vi "Operate.vi"(0 "Add in":refnum<class "Add.lvclass">, 11 "error in (no error)":errorcluster) -> (4 "Add out":refnum<class "Add.lvclass">, 15 "error out":errorcluster)   [LabVIEW 2020, in "Add.lvclass"]
uses:
  Add.lvclass
  C:/Users/khishore.kumar/Khishore/labview_tips_2024/src/Assignment 25/Arithmetic Operations/Arithmetic Operations.lvclass
  Arithmetic Operations.lvclass/Arithmetic Operations.ctl
  Accessors/Read/Read A.vi
  Accessors/Read/Read B.vi
  Accessors/Write/Write C.vi
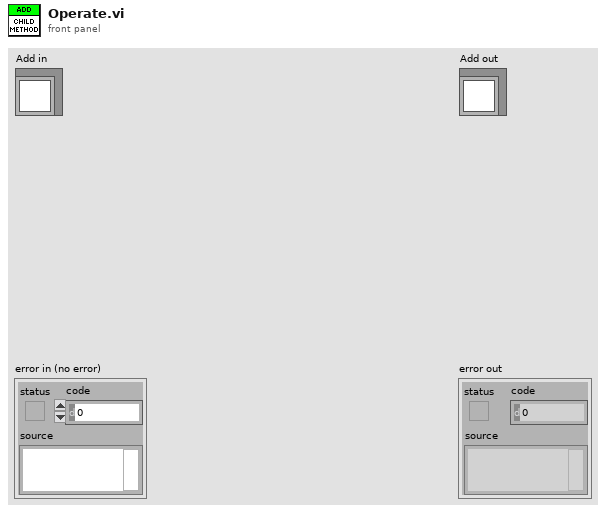
[diagram p1: front panel]
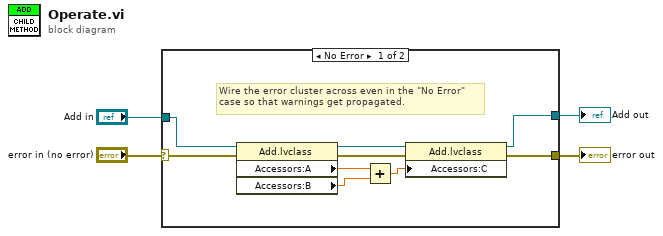
[diagram p0: block diagram]
diagram:
  n1 = case shown="No Error" "error in (no error)" {
    selector: "error in (no error)" -> [w12 w15]
    tunnel: [w5 w15] -> w3
    tunnel: [w6 w14] -> w1
    tunnel: "Add in" -> [w13 w14]
    frame No Error {
      # "Wire the error cluster across even in the \"No Error\"\ncase so that warnings get propagated."
      n2 = property class="Add.lvclass"(reference=w13, error in=w12) -> (reference out=w9:refnum<class "Add.lvclass">, error out=w8:errorcluster, "Accessors:A"=w11:dbl, "Accessors:B"=w10:dbl)
      n3 = Add(x=w11, y=w10) -> (x+y=w7:dbl)
      n4 = property class="Add.lvclass"(reference=w9, error in=w8, "Accessors:C"=w7) -> (reference out=w6:refnum<class "Add.lvclass">, error out=w5:errorcluster)
    }
    frame Error {
    }
  }
  "error out" <- w3
  "Add out" <- w1
